vi "运维调试界面.vi"() -> ()   [LabVIEW 2016, in "质控单元V4.lvlib"]
uses:
  <vilib>/Utility/miscctls.llb/LVPointTypeDef.ctl
  <vilib>/ptbypt/NI_PtbyPt.lvlib
panel:
  in  "数值":u8
  in  "向前寻道按钮":bool
  in  "向后寻道按钮":bool
  out "质控状态 4":T1
  out "质控状态 3":T1
  out "质控状态 2":T1
  out "质控状态":T1
  out "权限等级":string
  in  "布尔":bool
  in  "ZK定时设置":cluster{"启动":bool, "控制命令":T2, "测量参数":T3}(xcontrol)
  out "模块版本号":string
  in  "停止":bool
  in  "参数设置":bool
  in  "连接设置":bool
  in  "调试界面":bool
  in  "加标回收":bool
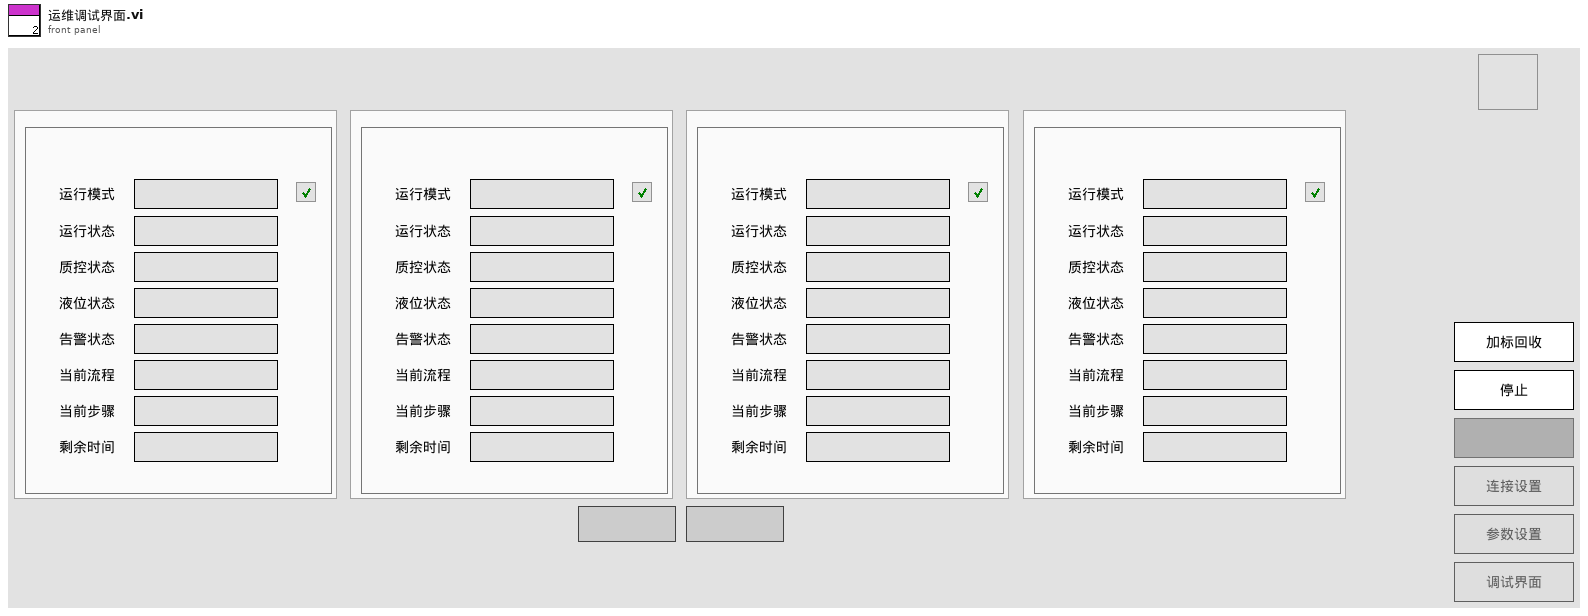
[diagram p1: front panel]
types:
  T1 = typedef "质控单元V4.lvlib/质控状态.ctl" = cluster{"模块名称":string, "通讯状态":bool, "运行模式":string, "运行状态":string, "质控状态":string, "液位状态":string, "告警状态":string, "当前流程":string, "当前步骤":string, "剩余时间":string}
  T2 = typedef "ZK定时设置.xctl/国标控制命令.ctl" = enum16{"加标回收（启动采配水）", "加标回收（不启动采配水）", "水样测试（启动采配水）", "水样测试（不启动采配水）"}
  T3 = typedef "ZK定时设置.xctl/测量参数.ctl" = cluster{"氨氮":bool, "总磷":bool, "总氮":bool, "CODMn":bool, "CODCr":bool}
  T4 = typedef "质控单元V4.lvlib/数据流类型.ctl" = cluster{"cmd":enum16{"start", "stop"}, "data":variant}
  T5 = typedef "LVPointTypeDef.ctl" = cluster{"Horizontal":i16, "Vertical":i16}
  T6 = typedef "质控单元V4.lvlib/质控仪器状态显示.ctl" = cluster{"运行模式":string, "运行状态":string, "液位状态":string, "告警状态":string, "当前流程":string, "当前步骤":string, "剩余时间":string}
  T7 = cluster{"氨氮":bool, "总磷":bool, "总氮":bool, "CODMn":bool, "CODCr":bool, "氨氮总磷":bool, "总磷总氮":bool}
  T8 = cluster{"启用参数选择":cluster{"氨氮启用":bool, "总磷启用":bool, "总氮启用":bool, "CODMn启用":bool, "CODCr启用":bool}, "流程":enum16{"加标回收（启动采配水）", "加标回收（不启动采配水）", "水样测试（启动采配水）", "水样测试（不启动采配水）"}}
  T9 = cluster{"氨氮启用":bool, "总磷启用":bool, "总氮启用":bool, "CODMn启用":bool, "CODCr启用":bool}
  T10 = enum16{"加标回收（启动采配水）", "加标回收（不启动采配水）", "水样测试（启动采配水）", "水样测试（不启动采配水）"}
  T11 = enum8{"Enabled", "Disabled", "Disabled and Grayed Out"}
  T12 = cluster{"Major":u16, "Minor":u16, "Fix":u16, "Build":u16}
  T13 = cluster{"氨氮":bool, "总磷":bool, "总氮":bool, "CODMn":bool, "CODCr":bool}
  T14 = enum32{"Bad", "Idle", "Run top level", "Running"}
  T15 = cluster{"启动参数":cluster{"氨氮启用":bool, "总磷启用":bool, "总氮启用":bool, "CODMn启用":bool, "CODCr启用":bool}, "流程参数":enum16{"加标回收（启动采配水）", "加标回收（不启动采配水）", "水样测试（启动采配水）", "水样测试（不启动采配水）"}}
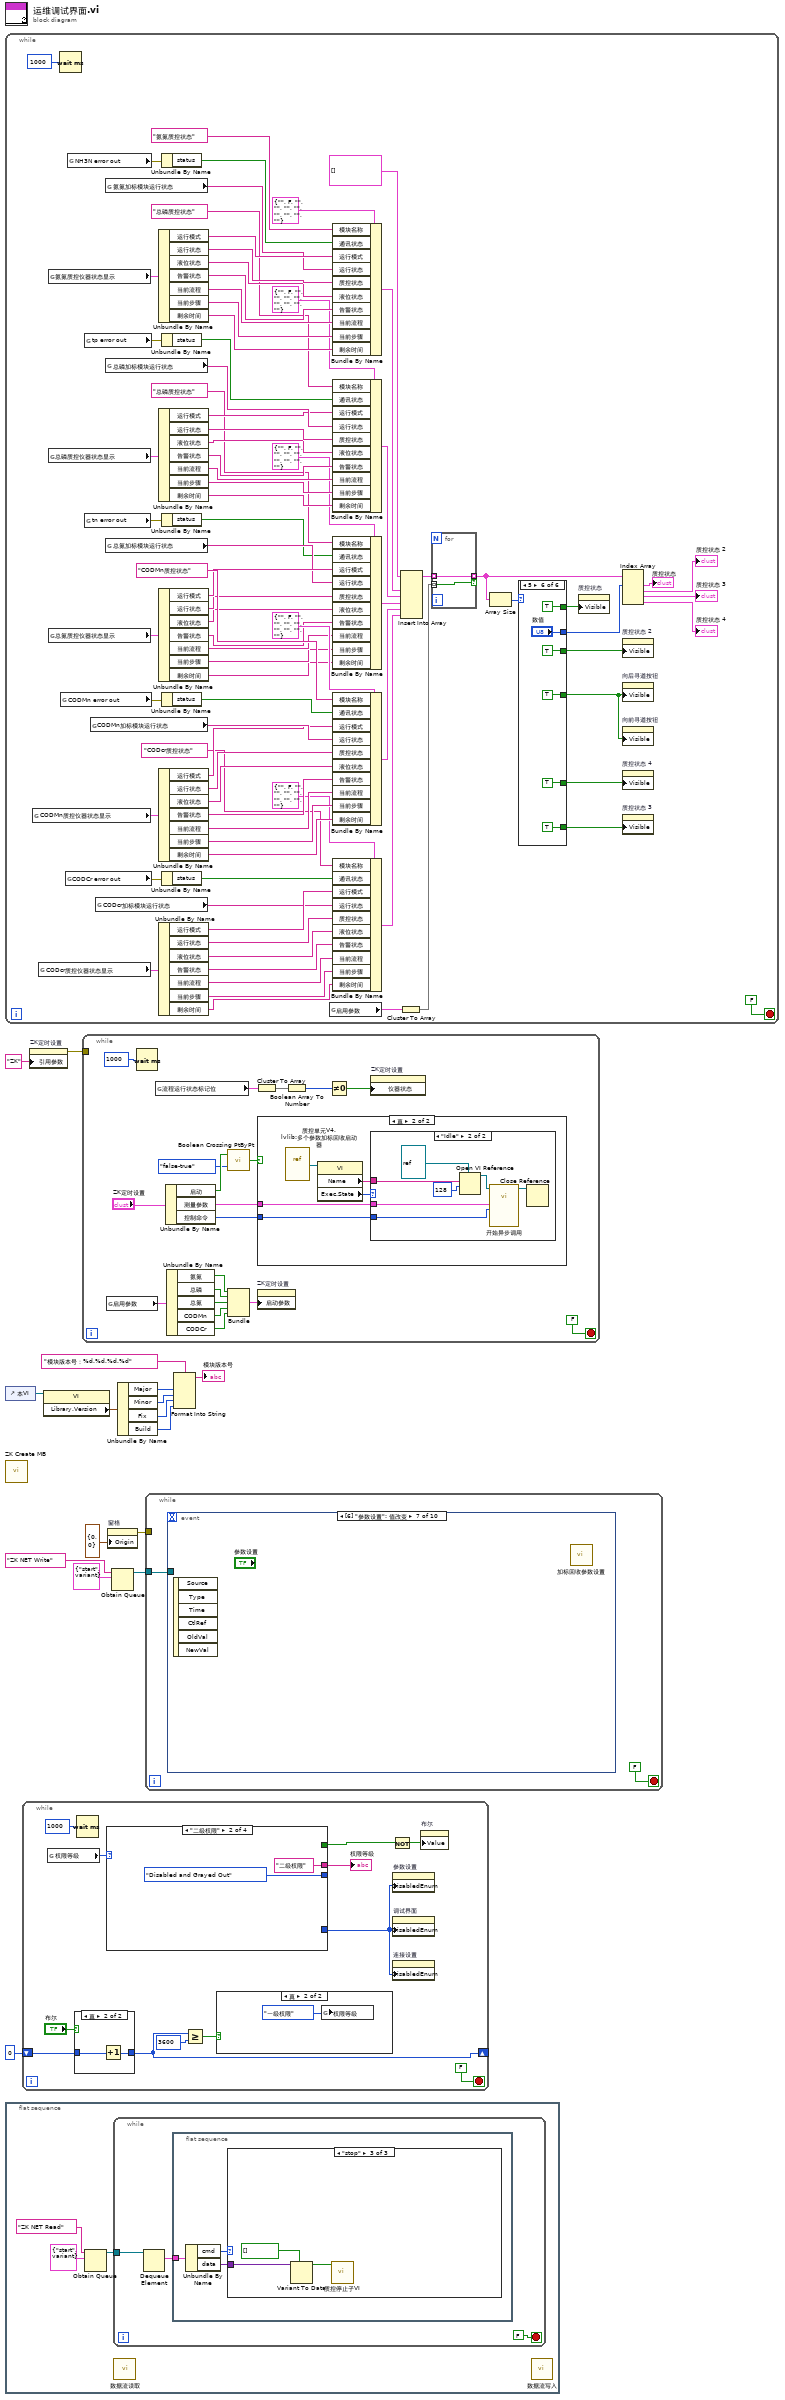
[diagram p0: block diagram]
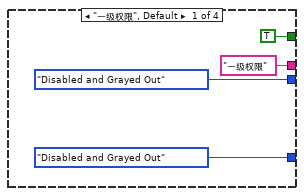
[diagram p2: hidden frame]
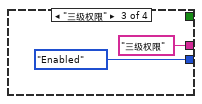
[diagram p3: hidden frame]
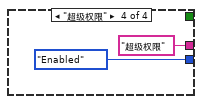
[diagram p4: hidden frame]
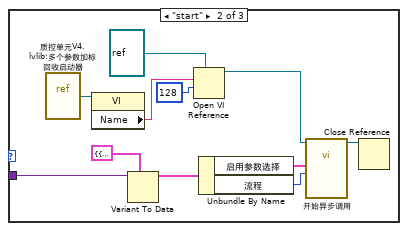
[diagram p8: hidden frame]
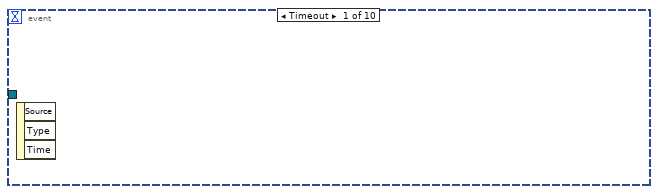
[diagram p11: hidden frame]
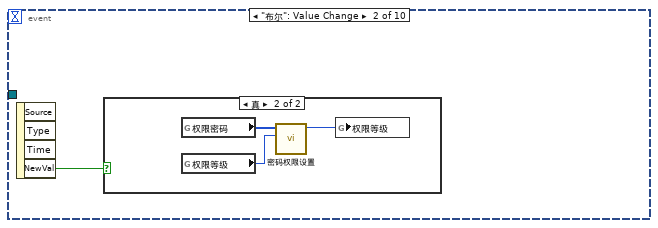
[diagram p12: hidden frame]
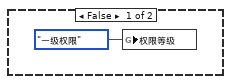
[diagram p13: hidden frame]
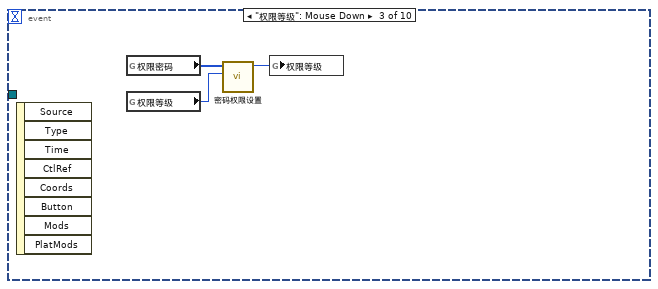
[diagram p14: hidden frame]
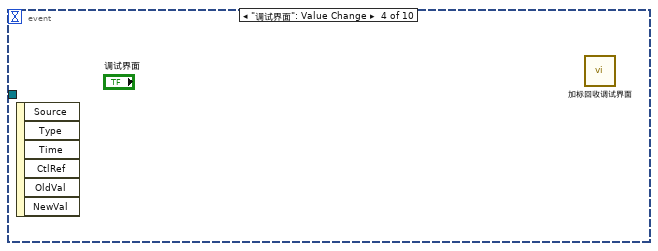
[diagram p15: hidden frame]
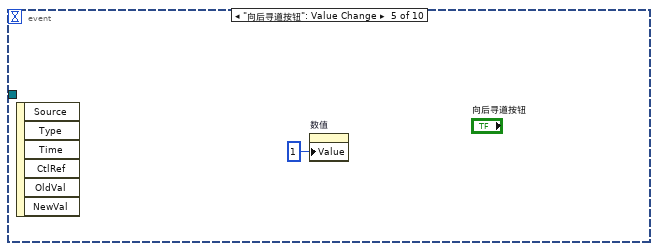
[diagram p16: hidden frame]
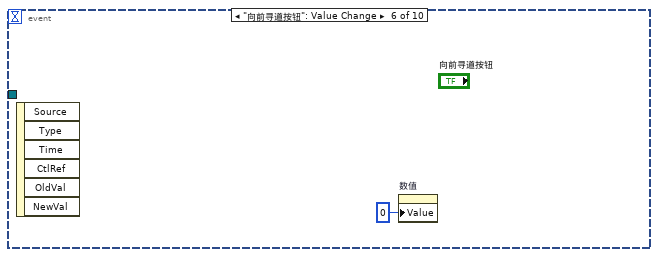
[diagram p17: hidden frame]
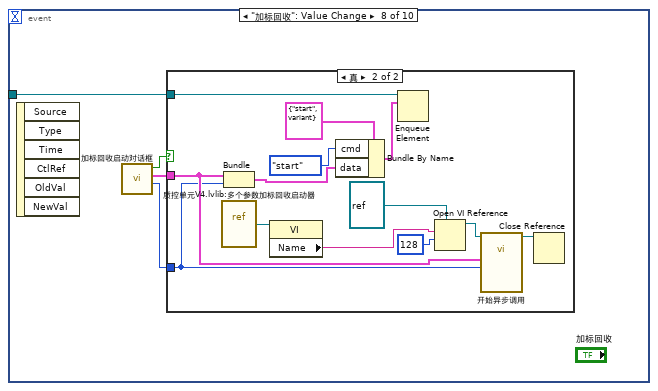
[diagram p18: hidden frame]
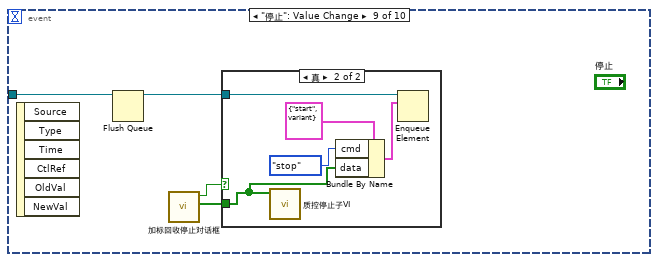
[diagram p20: hidden frame]
diagram:
  n1 = while {
    stop <- FALSE stop-if-true
    n2 = global read "ZK非断电保存全局变量.vi" "CODMn质控仪器状态显示"() -> (w97:T6)
    n3 = global read "ZK非断电保存全局变量.vi" "CODcr质控仪器状态显示"() -> (w34:T6)
    n4 = global read "ZK非断电保存全局变量.vi" "氨氮质控仪器状态显示"() -> (w100:T6)
    n5 = global read "ZK非断电保存全局变量.vi" "总磷质控仪器状态显示"() -> (w99:T6)
    n6 = global read "ZK非断电保存全局变量.vi" "总氮质控仪器状态显示"() -> (w98:T6)
    n7 = Wait (ms)(milliseconds to wait=u32 1000 ("等待时间（毫秒）")) -> ()  [unwired: 1 out]
    n8 = global read "ZK非断电保存全局变量.vi" "CODMn error out"() -> (w102:errorcluster)
    n9 = global read "ZK非断电保存全局变量.vi" "CODCr error out"() -> (w33:errorcluster)
    n10 = global read "ZK非断电保存全局变量.vi" "NH3N error out"() -> (w101:errorcluster)
    n11 = global read "ZK非断电保存全局变量.vi" "tp error out"() -> (w96:errorcluster)
    n12 = global read "ZK非断电保存全局变量.vi" "tn error out"() -> (w95:errorcluster)
    n13 = global read "ZK非断电保存全局变量.vi" "CODMn加标模块运行状态"() -> (w69:string)
    n14 = global read "ZK非断电保存全局变量.vi" "CODcr加标模块运行状态"() -> (w38:string)
    n15 = global read "ZK非断电保存全局变量.vi" "氨氮加标模块运行状态"() -> (w90:string)
    n16 = global read "ZK非断电保存全局变量.vi" "总磷加标模块运行状态"() -> (w82:string)
    n17 = global read "ZK非断电保存全局变量.vi" "总氮加标模块运行状态"() -> (w58:string)
    n18 = Unbundle By Name(w100) -> ("运行模式"=w91:string, "运行状态"=w89:string, "液位状态"=w88:string, "告警状态"=w87:string, "当前流程"=w86:string, "当前步骤"=w85:string, "剩余时间"=w84:string)
    n19 = Unbundle By Name(w99) -> ("运行模式"=w81:string, "运行状态"=w80:string, "液位状态"=w79:string, "告警状态"=w78:string, "当前流程"=w77:string, "当前步骤"=w76:string, "剩余时间"=w75:string)
    n20 = Unbundle By Name(w98) -> ("运行模式"=w59:string, "运行状态"=w56:string, "液位状态"=w55:string, "告警状态"=w54:string, "当前流程"=w53:string, "当前步骤"=w52:string, "剩余时间"=w51:string)
    n21 = Unbundle By Name(w97) -> ("运行模式"=w68:string, "运行状态"=w67:string, "液位状态"=w66:string, "告警状态"=w65:string, "当前流程"=w64:string, "当前步骤"=w63:string, "剩余时间"=w62:string)
    n22 = Unbundle By Name(w34) -> ("运行模式"=w39:string, "运行状态"=w40:string, "液位状态"=w41:string, "告警状态"=w42:string, "当前流程"=w43:string, "当前步骤"=w44:string, "剩余时间"=w45:string)
    n23 = Unbundle By Name(w101) -> ("status"=w93:bool)
    n24 = Unbundle By Name(w96) -> ("status"=w73:bool)
    n25 = Unbundle By Name(w95) -> ("status"=w57:bool)
    n26 = Unbundle By Name(w102) -> ("status"=w70:bool)
    n27 = Unbundle By Name(w33) -> ("status"=w37:bool)
    n28 = global read "ZK断电保存全局变量.vi" "启用参数"() -> (w30:T7)
    n29 = Bundle By Name(cluster=T1 {"模块名称"="", "通讯状态"=FALSE, "运行模式"="", "运行状态"="", "质控状态"="", "液位状态"="", "告警状态"="", "当前流程"="", "当前步骤"="", "剩余时间"=""} ("质控状态"), "模块名称"="氨氮质控状态", "通讯状态"=w93, "运行模式"=w91, "运行状态"=w90, "质控状态"=w89, "液位状态"=w88, "告警状态"=w87, "当前流程"=w86, "当前步骤"=w85, "剩余时间"=w84) -> (w50:T1)
    n30 = Bundle By Name(cluster=T1 {"模块名称"="", "通讯状态"=FALSE, "运行模式"="", "运行状态"="", "质控状态"="", "液位状态"="", "告警状态"="", "当前流程"="", "当前步骤"="", "剩余时间"=""} ("质控状态"), "模块名称"="总磷质控状态", "通讯状态"=w73, "运行模式"=w81, "运行状态"=w82, "质控状态"=w80, "液位状态"=w79, "告警状态"=w78, "当前流程"=w77, "当前步骤"=w76, "剩余时间"=w75) -> (w48:T1)
    n31 = Bundle By Name(cluster=T1 {"模块名称"="", "通讯状态"=FALSE, "运行模式"="", "运行状态"="", "质控状态"="", "液位状态"="", "告警状态"="", "当前流程"="", "当前步骤"="", "剩余时间"=""} ("质控状态"), "模块名称"="总磷质控状态", "通讯状态"=w57, "运行模式"=w59, "运行状态"=w58, "质控状态"=w56, "液位状态"=w55, "告警状态"=w54, "当前流程"=w53, "当前步骤"=w52, "剩余时间"=w51) -> (w47:T1)
    n32 = Bundle By Name(cluster=T1 {"模块名称"="", "通讯状态"=FALSE, "运行模式"="", "运行状态"="", "质控状态"="", "液位状态"="", "告警状态"="", "当前流程"="", "当前步骤"="", "剩余时间"=""} ("质控状态"), "模块名称"="CODMn质控状态", "通讯状态"=w70, "运行模式"=w68, "运行状态"=w69, "质控状态"=w67, "液位状态"=w66, "告警状态"=w65, "当前流程"=w64, "当前步骤"=w63, "剩余时间"=w62) -> (w46:T1)
    n33 = Bundle By Name(cluster=T1 {"模块名称"="", "通讯状态"=FALSE, "运行模式"="", "运行状态"="", "质控状态"="", "液位状态"="", "告警状态"="", "当前流程"="", "当前步骤"="", "剩余时间"=""} ("质控状态"), "模块名称"="CODcr质控状态", "通讯状态"=w37, "运行模式"=w39, "运行状态"=w38, "质控状态"=w40, "液位状态"=w41, "告警状态"=w42, "当前流程"=w43, "当前步骤"=w44, "剩余时间"=w45) -> (w32:T1)
    n34 = Cluster To Array(cluster=w30) -> (array=w29:bool[])
    n35 = Insert Into Array(array=T1[] [] ("数组"), new element #1=w50, new element #2=w48, new element #3=w47, new element #4=w46, new element #5=w32) -> (w31:T1[])  [unwired: 1 in]
    n36 = for {
      tunnel: w31 -> [w126] mode=indexing
      tunnel: w29 -> [w125] mode=indexing
      tunnel: [w126] -> w24 mode=indexing if=w125
    }
    n37 = Array Size(array=w24) -> (size(s)=w23:i32)
    n38 = case shown="5" w23 {
      tunnel: [FALSE TRUE TRUE TRUE TRUE TRUE] -> w22
      tunnel: [FALSE _ TRUE TRUE TRUE TRUE] -> w21
      tunnel: [FALSE _ _ TRUE TRUE TRUE] -> w20
      tunnel: [FALSE _ _ _ TRUE TRUE] -> w19
      tunnel: [_ _ _ _ _ TRUE] -> w18
      tunnel: [_ _ _ _ _ "数值"] -> w17
      frame 0, Default {
      }
      frame 1 {
      }
      frame 2 {
      }
      frame 3 {
      }
      frame 4 {
      }
      frame 5 {
      }
    }
    n39 = property on="质控状态" class="Clust (严格)"("Visible"=w22) -> ()  [unwired: 2 in, 2 out]
    n40 = Index Array(array=w24, index #1=w17) -> (element #1=→"质控状态":T1, element #2=→"质控状态 2":T1, element #3=→"质控状态 3":T1, element #4=→"质控状态 4":T1)  [unwired: 3 in]
    n41 = property on="质控状态 2" class="Clust (严格)"("Visible"=w21) -> ()  [unwired: 2 in, 2 out]
    n42 = property on="向后寻道按钮" class="Bool"("Visible"=w18) -> ()  [unwired: 2 in, 2 out]
    n43 = property on="向前寻道按钮" class="Bool"("Visible"=w18) -> ()  [unwired: 2 in, 2 out]
    n44 = property on="质控状态 4" class="Clust (严格)"("Visible"=w19) -> ()  [unwired: 2 in, 2 out]
    n45 = property on="质控状态 3" class="Clust (严格)"("Visible"=w20) -> ()  [unwired: 2 in, 2 out]
  }
  n46 = control-ref of="本VI"() -> (w14:refnum<vi>)
  n47 = call "ZK Create MB.vi"() -> ()  [unwired: 12 in]
  n48 = flat-sequence {
    frame #0 {
      n49 = Obtain Queue(name (unnamed)="ZK NET Read" ("名称（未命名）"), element data type=T4 {"cmd"=enum."start", "data"=variant} ("簇")) -> (queue out=w128:refnum<queue>)  [unwired: 3 in, 2 out]
      n50 = while {
        tunnel: w128 -> [w132]
        stop <- FALSE stop-if-true
        n51 = Dequeue Element(queue=w132) -> (element=w130:T4)  [unwired: 2 in, 3 out]
        n52 = flat-sequence {
          tunnel: w130 -> [w135]
          frame #0 {
            n53 = Unbundle By Name(w135) -> ("cmd"=w134:enum16{"start", "stop"}, "data"=w133:variant)
            n54 = case shown="\"stop\"" w134 {
              tunnel: w133 -> [_ w140 w149]
              frame Default {
              }
              frame "start" {
                n55 = vi-ref "质控单元V4.lvlib:多个参数加标回收启动器.vi"() -> (w146:refnum<vi>)
                n56 = property class="VI"(reference=w146) -> ("Name"=w145:string)  [unwired: 1 in, 2 out]
                n57 = Variant To Data(type=T8 {"启用参数选择"={"氨氮启用"=FALSE, "总磷启用"=FALSE, "总氮启用"=FALSE, "CODMn启用"=FALSE, "CODCr启用"=FALSE}, "流程"=enum."加标回收（启动采配水）"} ("data"), Variant=w140) -> (data=w138:T8)  [unwired: 1 in, 1 out]
                n58 = Open VI Reference(type specifier VI Refnum (for type only)=refnum<vi> refnum, vi path=w145, options=128 ("选项")) -> (vi reference=w143:refnum<vi>)  [unwired: 3 in, 1 out]
                n59 = Unbundle By Name(w138) -> ("启用参数选择"=w137:T9, "流程"=w136:T10)
                n60 = call-by-ref "开始异步调用"(reference=w143, "流程"=w136, "启用参数选择"=w137) -> (reference out=w142:refnum<vi>)  [unwired: 11 in, 1 out]
                n61 = Close Reference(reference=w142) -> ()  [unwired: 1 in, 1 out]
              }
              frame "stop" {
                n62 = Variant To Data(type=bool[] [] ("数组"), Variant=w149) -> (data=w147:bool[])  [unwired: 1 in, 1 out]
                n63 = call "质控停止子VI.vi"("数组"=w147) -> ()  [unwired: 11 in]
              }
            }
          }
        }
      }
      n64 = call "数据流读取.vi"() -> ()  [unwired: 12 in]
      n65 = call "数据流写入.vi"() -> ()  [unwired: 12 in]
    }
  }
  n66 = while {
    shift-right: [w160] -> _
    shift-left: 0 -> [w161]
    stop <- FALSE stop-if-true
    n67 = global read "ZK非断电保存全局变量.vi" "权限等级"() -> (w155:enum16{"一级权限", "二级权限", "三级权限", "超级权限"})
    n68 = case shown="真" "布尔" {
      tunnel: w161 -> [_ w174]
      tunnel: [_ w173] -> w160
      frame False {
      }
      frame True {
        n69 = Increment(x=w174) -> (x+1=w173:i32)
      }
    }
    n70 = Wait (ms)(milliseconds to wait=u32 1000 ("等待时间（毫秒）")) -> ()  [unwired: 1 out]
    n71 = case shown="\"二级权限\"" w155 {
      tunnel: [T11."Disabled and Grayed Out" ("禁用") _ _ _] -> w150
      tunnel: ["一级权限" "二级权限" "三级权限" "超级权限"] -> w153
      tunnel: [TRUE ("布尔") _ _ _] -> w152
      tunnel: [T11."Disabled and Grayed Out" ("禁用") T11."Disabled and Grayed Out" ("禁用") T11."Enabled" ("禁用") T11."Enabled" ("禁用")] -> _
      frame "一级权限", Default {
      }
      frame "二级权限" {
      }
      frame "三级权限" {
      }
      frame "超级权限" {
      }
    }
    "权限等级" <- w153
    n72 = Greater Or Equal?(x=w160, y=3600) -> (x >= y?=w158:bool)
    n73 = case shown="真" w158 {
      frame False {
      }
      frame True {
        n74 = global write "ZK非断电保存全局变量.vi" "权限等级"(enum16{"一级权限", "二级权限", "三级权限", "超级权限"}."一级权限" ("权限等级")) -> ()
      }
    }
    n75 = Not(x=w152) -> (.not. x?=w151:bool)
    n76 = property on="参数设置" class="Bool"("DisabledEnum"=w150) -> ()  [unwired: 2 in, 2 out]
    n77 = property on="调试界面" class="Bool"("DisabledEnum"=w150) -> ()  [unwired: 2 in, 2 out]
    n78 = property on="连接设置" class="Bool"("DisabledEnum"=w150) -> ()  [unwired: 2 in, 2 out]
    n79 = property on="布尔" class="Bool (严格)"("Value"=w151) -> ()  [unwired: 2 in, 2 out]
  }
  n80 = property on="ZK定时设置" class="ZK定时设置 (严格)"("引用参数"="ZK") -> (error out=w5:errorcluster)  [unwired: 2 in, 1 out]
  n81 = property class="VI"(reference=w14) -> ("Library.Version"=w13:T12)  [unwired: 1 in, 2 out]
  n82 = while {
    tunnel: w5 -> [_]
    stop <- FALSE stop-if-true
    n83 = global read "ZK断电保存全局变量.vi" "启用参数"() -> (w181:T7)
    n84 = Wait (ms)(milliseconds to wait=u32 1000 ("等待时间（毫秒）")) -> ()  [unwired: 1 out]
    n85 = global read "ZK非断电保存全局变量.vi" "流程运行状态标记位"() -> (w188:T7)
    n86 = Unbundle By Name("ZK定时设置") -> ("启动"=w184:bool, "测量参数"=w190:T3, "控制命令"=w189:T2)
    n87 = Unbundle By Name(w181) -> ("氨氮"=w180:bool, "总磷"=w179:bool, "总氮"=w178:bool, "CODMn"=w177:bool, "CODCr"=w176:bool)
    n88 = call <vilib>:"Boolean Crossing PtByPt.vi"("direction"=enum16{"either", "false-true", "true-false"}."false-true", "input"=w184) -> ("crossing"=w183:bool)  [unwired: 1 in]
    n89 = Bundle("氨氮"=w180, "总磷"=w179, "总氮"=w178, "CODMn"=w177, "CODCr"=w176) -> (w175:T13)  [unwired: 1 in]
    n90 = Cluster To Array(cluster=w188) -> (array=w187:bool[])
    n91 = case shown="真" w183 {
      tunnel: w190 -> [_ w196]
      tunnel: w189 -> [_ w195]
      frame False {
      }
      frame True {
        n92 = vi-ref "质控单元V4.lvlib:多个参数加标回收启动器.vi"() -> (w197:refnum<vi>)
        n93 = property class="VI"(reference=w197) -> ("Name"=w198:string, "Exec.State"=w194:T14)  [unwired: 1 in, 2 out]
        n94 = case shown="\"Idle\"" w194 {
          tunnel: w198 -> [_ w201]
          tunnel: w196 -> [_ w200]
          tunnel: w195 -> [_ w199]
          frame "Bad", Default {
          }
          frame "Idle" {
            n95 = Open VI Reference(type specifier VI Refnum (for type only)=refnum<vi> refnum, vi path=w201, options=128 ("选项")) -> (vi reference=w203:refnum<vi>)  [unwired: 3 in, 1 out]
            n96 = call-by-ref "开始异步调用"(reference=w203, "流程"=w199, "启用参数选择"=w200) -> (reference out=w204:refnum<vi>)  [unwired: 11 in, 1 out]
            n97 = Close Reference(reference=w204) -> ()  [unwired: 1 in, 1 out]
          }
        }
      }
    }
    n98 = property on="ZK定时设置" class="ZK定时设置 (严格)"("启动参数"=w175) -> ()  [unwired: 2 in, 2 out]
    n99 = Boolean Array To Number(Boolean array=w187) -> (number=w186:u32)
    n100 = Not Equal To 0?(x=w186) -> (x != 0?=w185:bool)
    n101 = property on="ZK定时设置" class="ZK定时设置 (严格)"("仪器状态"=w185) -> ()  [unwired: 2 in, 2 out]
  }
  n102 = property on="窗格" class="Pane"("Origin"=T5 {"Horizontal"=0, "Vertical"=0} ("原点")) -> (error out=w15:errorcluster)  [unwired: 2 in, 1 out]
  n103 = Obtain Queue(name (unnamed)="ZK NET Write" ("名称（未命名）"), element data type=T4 {"cmd"=enum."start", "data"=variant} ("簇")) -> (queue out=w3:refnum<queue>)  [unwired: 3 in, 2 out]
  n104 = Unbundle By Name(w13) -> ("Major"=w11:u16, "Minor"=w10:u16, "Fix"=w9:u16, "Build"=w8:u16)
  n105 = while {
    tunnel: w15 -> [_]
    tunnel: w3 -> [w206]
    stop <- FALSE stop-if-true
    n106 = event shown="[6] \"参数设置\": 值改变" {
      selector: _ -> [_ _ _ _ _ _ _ _ _ _]
      dyn-events: _ -> [_ _ _ _ _ _ _ _ _ _]
      timeout: _ -> [_ _ _ _ _ _ _ _ _ _]
      tunnel: w206 -> [_ _ _ _ _ _ _ w218 w238 _]
      event Timeout {
        n107 = event-data() -> ()  [unwired: 1 in, 3 out]
      }
      event "布尔": Value Change {
        n108 = event-data() -> ("NewVal"=w208:bool)  [unwired: 1 in, 3 out]
        n109 = case shown="真" w208 {
          frame False {
            n110 = global write "ZK非断电保存全局变量.vi" "权限等级"(enum16{"一级权限", "二级权限", "三级权限", "超级权限"}."一级权限" ("权限等级")) -> ()
          }
          frame True {
            n111 = global read "ZK非断电保存全局变量.vi" "权限密码"() -> (w212:u32[])
            n112 = global read "ZK非断电保存全局变量.vi" "权限等级"() -> (w210:enum16{"一级权限", "二级权限", "三级权限", "超级权限"})
            n113 = call "密码权限设置.vi"("权限输入"=w210, "权限密码"=w212) -> ("权限输出"=w211:enum16{"一级权限", "二级权限", "三级权限", "超级权限"})  [unwired: 9 in]
            n114 = global write "ZK非断电保存全局变量.vi" "权限等级"(w211) -> ()
          }
        }
      }
      event "权限等级": Mouse Down {
        n115 = event-data() -> ()  [unwired: 1 in, 8 out]
        n116 = global read "ZK非断电保存全局变量.vi" "权限密码"() -> (w215:u32[])
        n117 = global read "ZK非断电保存全局变量.vi" "权限等级"() -> (w213:enum16{"一级权限", "二级权限", "三级权限", "超级权限"})
        n118 = call "密码权限设置.vi"("权限输入"=w213, "权限密码"=w215) -> ("权限输出"=w214:enum16{"一级权限", "二级权限", "三级权限", "超级权限"})  [unwired: 9 in]
        n119 = global write "ZK非断电保存全局变量.vi" "权限等级"(w214) -> ()
      }
      event "调试界面": Value Change {
        n120 = event-data() -> ()  [unwired: 1 in, 6 out]
        n121 = call "加标回收调试界面.vi"() -> ()  [unwired: 12 in]
      }
      event "向后寻道按钮": Value Change {
        n122 = event-data() -> ()  [unwired: 1 in, 6 out]
        n123 = property on="数值" class="DigNum (严格)"("Value"=u8 1 ("数值")) -> ()  [unwired: 2 in, 2 out]
      }
      event "向前寻道按钮": Value Change {
        n124 = event-data() -> ()  [unwired: 1 in, 6 out]
        n125 = property on="数值" class="DigNum (严格)"("Value"=u8 0 ("数值")) -> ()  [unwired: 2 in, 2 out]
      }
      event "参数设置": Value Change {
        n126 = event-data() -> ()  [unwired: 1 in, 6 out]
        n127 = call "加标回收参数设置.vi"() -> ()  [unwired: 12 in]
      }
      event "加标回收": Value Change {
        n128 = event-data() -> ()  [unwired: 1 in, 6 out]
        n129 = call "加标回收启动对话框.vi"() -> ("流程参数"=w219:T10, "启动参数"=w220:T9, "check ？"=w221:bool)  [unwired: 9 in]
        n130 = case shown="真" w221 {
          tunnel: w220 -> [_ w227]
          tunnel: w219 -> [_ w226]
          tunnel: w218 -> [_ w228]
          frame False {
          }
          frame True {
            n131 = vi-ref "质控单元V4.lvlib:多个参数加标回收启动器.vi"() -> (w234:refnum<vi>)
            n132 = Bundle("启动参数"=w227, "流程参数"=w226) -> (w223:T15)  [unwired: 1 in]
            n133 = property class="VI"(reference=w234) -> ("Name"=w233:string)  [unwired: 1 in, 2 out]
            n134 = Bundle By Name(cluster=T4 {"cmd"=enum."start", "data"=variant} ("簇"), "cmd"=enum16{"start", "stop"}."start", "data"=w223) -> (w222:T4)
            n135 = Enqueue Element(queue=w228, element=w222) -> ()  [unwired: 2 in, 3 out]
            n136 = Open VI Reference(type specifier VI Refnum (for type only)=refnum<vi> refnum, vi path=w233, options=128 ("选项")) -> (vi reference=w231:refnum<vi>)  [unwired: 3 in, 1 out]
            n137 = call-by-ref "开始异步调用"(reference=w231, "流程"=w226, "启用参数选择"=w227) -> (reference out=w230:refnum<vi>)  [unwired: 11 in, 1 out]
            n138 = Close Reference(reference=w230) -> ()  [unwired: 1 in, 1 out]
          }
        }
      }
      event "停止": Value Change {
        n139 = event-data() -> ()  [unwired: 1 in, 6 out]
        n140 = Flush Queue(queue=w238) -> (queue out=w237:refnum<queue>)  [unwired: 1 in, 2 out]
        n141 = call "加标回收停止对话框.vi"() -> ("数组"=w236:bool[], "check？"=w235:bool)  [unwired: 10 in]
        n142 = case shown="真" w235 {
          tunnel: w237 -> [_ w243]
          tunnel: w236 -> [_ w239]
          frame False {
          }
          frame True {
            n143 = call "质控停止子VI.vi"("数组"=w239) -> ()  [unwired: 11 in]
            n144 = Bundle By Name(cluster=T4 {"cmd"=enum."start", "data"=variant} ("簇"), "cmd"=enum16{"start", "stop"}."stop", "data"=w239) -> (w240:T4)
            n145 = Enqueue Element(queue=w243, element=w240) -> ()  [unwired: 2 in, 3 out]
          }
        }
      }
      event "连接设置": Value Change {
        n146 = event-data() -> ()  [unwired: 1 in, 6 out]
        n147 = call "串口配置.vi"() -> ()  [unwired: 12 in]
      }
    }
  }
  n148 = Format Into String(format string="模块版本号：%d.%d.%d.%d" ("格式字符串"), w11, w10, w9, w8) -> (resulting string=→"模块版本号":string)  [unwired: 2 in, 1 out]
